vi "Stepper RT Solution Rev B.vi"() -> ()   [LabVIEW 2014]
uses:
  <vilib>/rvi/interface/nirviOpenFPGA/nirviOpenFPGA.xnode
  <vilib>/rvi/interface/nirviCloseFPGA/nirviCloseFPGA.xnode
  <vilib>/rvi/interface/nirviReadWriteControl/nirviReadWriteControl.xnode
  <vilib>/FPGAPlugInAG/Dynamic/niLvFpga_Close_Dynamic.vi
  NiFpgaLv.dll
  <vilib>/Utility/error.llb/Error Cluster From Error Code.vi
  <vilib>/rvi/interface/Simulation/niFpgaSimulationCallBeginRW.vi
  <vilib>/rvi/errors/niLvFpgaAdjustHostInterfaceError.vi
  FPGA Bitfiles/MotorLabAProject_FPGATarget_StepperFPGARevB_tJXaSwyGK8w.lvbitx
  Stepper FPGA Rev B.vi
  <vilib>/FPGAPlugInAG/cRIO-9074/niLvFpga_Open_cRIO-9074.vi
  <vilib>/rvi/interface/common/dynamic/niFpgaDynamicAddResources.vi
panel:
  out "Current (Steps)":i32
  out "Steps to move":i32
  in  "Reset Step Counter":bool
  in  "stop":bool
  in  "Stepper Command (Deg)":dbl(knob)
  # "Run Stepper FGGA Rev B. VI first,\nset its stpe period to 2000, then run this \nVI."
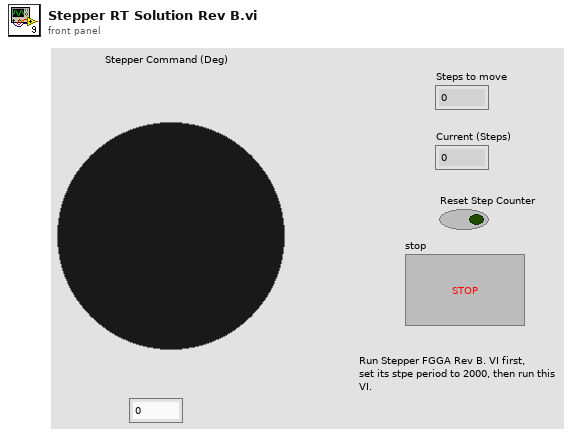
[diagram p1: front panel]
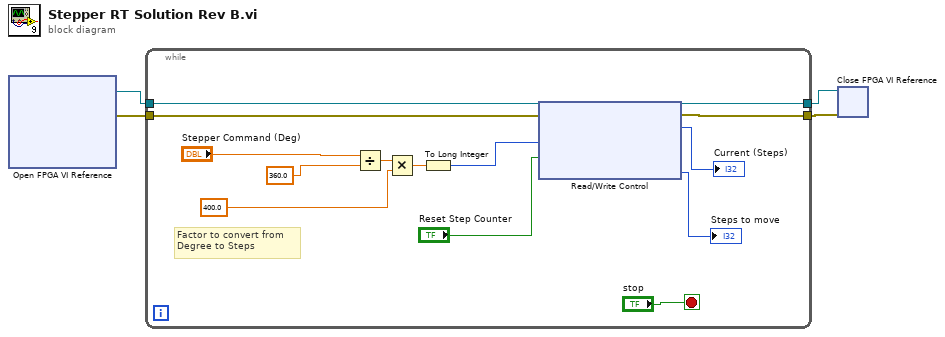
[diagram p0: block diagram]
diagram:
  n1 = xnode "Open FPGA VI Reference"() -> ("FPGA VI Reference Out"=w4:refnum<k20>, "error out"=w3:errorcluster)  [unwired: 2 in]
  n2 = while {
    tunnel: w4 -> [w18]
    tunnel: w3 -> [w17]
    tunnel: [w16] -> w2
    tunnel: [w15] -> w1
    stop <- "stop" stop-if-true
    # "Factor to convert from \nDegree to Steps"
    n3 = Divide(x="Stepper Command (Deg)", y=360.0) -> (x/y=w14:dbl)
    n4 = Multiply(x=w14, y=400.0) -> (x*y=w11:dbl)
    n5 = To Long Integer(number=w11) -> (32bit integer=w8:i32)
    n6 = xnode "Read/Write Control"("FPGA VI Reference In"=w18, "error in"=w17, "Desired Position (Steps)"=w8, "Reset Step Counter"="Reset Step Counter") -> ("FPGA VI Reference Out"=w16:refnum<k20>, "error out"=w15:errorcluster, "Current (Steps)"=→"Current (Steps)":i32, "Steps to move"=→"Steps to move":i32)
  }
  n7 = xnode "Close FPGA VI Reference"("FPGA VI Reference In"=w2, "error in"=w1) -> ()  [unwired: 1 out]
